vi "Preview.vi"(8 "error in (no error)":errorcluster, 10 "collect dependencies? (F)":bool, 11 "Build in":refnum<class "NI_AB_API_Build.lvclass">) -> (0 "error out":errorcluster, 1 "Dependencies":T1[](array[typedef]), 2 "GeneratedFiles":path[](array[path]), 3 "Build out":refnum<class "NI_AB_API_Build.lvclass">)   [LabVIEW 2020, in "NI_AB_API_Build.lvclass"]
uses:
  <vilib>/AppBuilder/AB_API/Build/NI_AB_API_Build.lvclass
  <vilib>/AppBuilder/AB_Dependency.ctl
  <vilib>/Utility/lvfile.llb/LVFileType.ctl
  <vilib>/AppBuilder/AB_API/Build/NI_AB_API_Build.lvclass/NI_AB_API_Build.ctl
  <vilib>/Utility/lvfile.llb/NI_FileType.lvlib
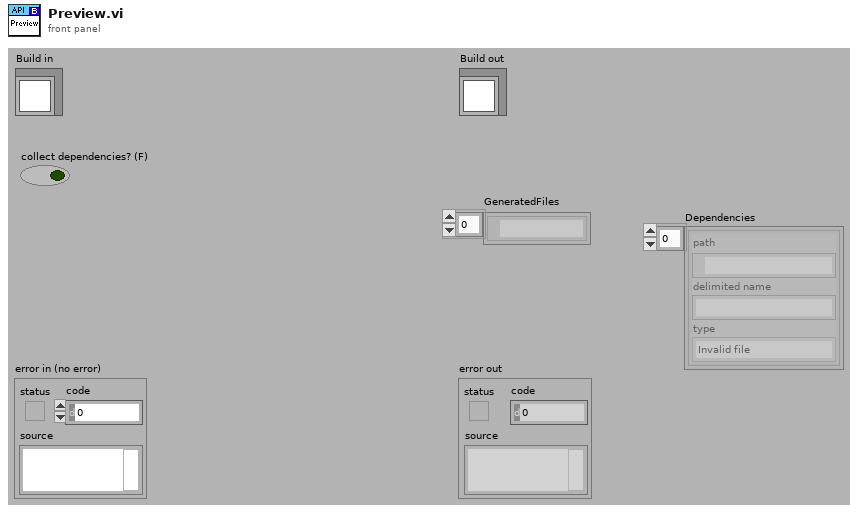
[diagram p1: front panel]
types:
  T1 = typedef "AB_Dependency.ctl" = cluster{"path":path, "delimited name":string, "type":T2}
  T2 = typedef "NI_FileType.lvlib/LVFileType.ctl" = enum32{"Invalid file", "Unknown type", "Instrument", "Control", "Polymorphic VI", "Project", "Library", "LVClass", "XControl", "XNode", "Shared library", ".NET assembly", "ActiveX interface", "CIN", "Run-time menu", "Palette menu", "Help file", "LLB", "XNode Edit Dependency", "Class Private Data Control", "Statechart", "MathScript .m file", "Ladder Diagram", "LVLibp", "XNode Build Dependency"}
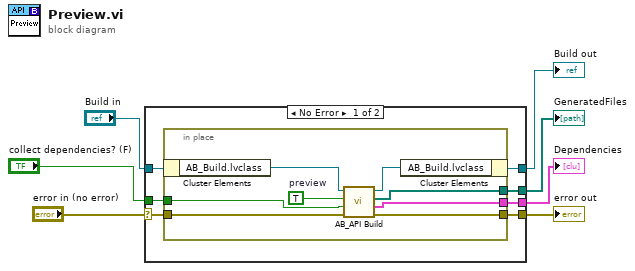
[diagram p0: block diagram]
diagram:
  n1 = case shown="No Error" "error in (no error)" {
    selector: "error in (no error)" -> [w13 w24]
    tunnel: [w12 w24] -> w6
    tunnel: [w10 w23] -> w4
    tunnel: "Build in" -> [w11 w23]
    tunnel: [w14 _] -> w3
    tunnel: [w9 _] -> w2
    tunnel: "collect dependencies? (F)" -> [w8 _]
    frame No Error {
      n2 = in-place {
        in-place-border: [w22] -> w14
        in-place-border: w13 -> [w21]
        in-place-border: [w20] -> w12
        in-place-border: [w16] -> w9
        in-place-border: w8 -> [w15]
        w19 = TRUE  # preview
        n3 = in-place-cluster #1(w11) -> ("AB_Build.lvclass"=w18:refnum<class "AB_Build.lvclass">)
        n4 = call <vilib>:"AB_API Build.vi"("error in (no error)"=w21, "collect dependencies?"=w15, "preview"=w19, "Build in"=w18) -> ("error out"=w20:errorcluster, "Dependencies"=w16:T1[], "GeneratedFiles"=w22:path[], "Build out"=w17:refnum<class "AB_Build.lvclass">)  [unwired: 4 out]
        n5 = in-place-cluster #1("AB_Build.lvclass"=w17) -> (w10:refnum<class "NI_AB_API_Build.lvclass">)
      }
    }
    frame Error {
    }
  }
  "error out" <- w6
  "Build out" <- w4
  "GeneratedFiles" <- w3
  "Dependencies" <- w2
